vi "Launch Dialog Box.vi"(8 "error in (no error)":errorcluster, 10 "DialogBox":refnum<class "IDialogBox.lvclass">, 11 "IDialogBox in":refnum<class "IDialogBox.lvclass">) -> (0 "error out":errorcluster, 3 "IDialogBox out":refnum<class "IDialogBox.lvclass">)   [LabVIEW 2015, in "IDialogBox.lvlib" / "IDialogBox.lvclass"]
doc: "<License>\nCopyright © 2017 Composed Systems, LLC | All rights reserved\nwww.composed.io\n\nAuthor: Ethan Stern <ethan.stern@composed.io>\n\nThis software is provided \"AS IS\" WITHOUT WARRANTIES, either express or implied, AND IS FOR EDUCATIONAL PURPOSES ONLY.\n</License>"
uses:
  IDialogBox.lvclass
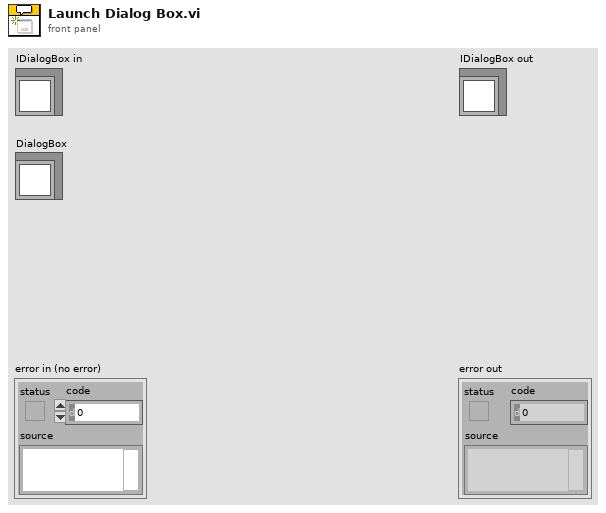
[diagram p1: front panel]
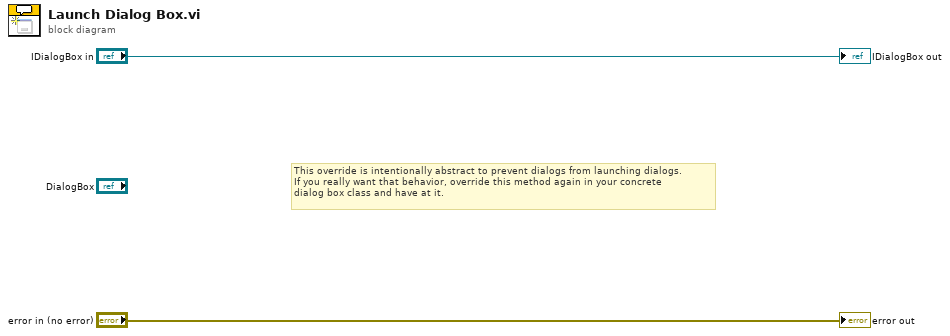
[diagram p0: block diagram]
diagram:
  # "This override is intentionally abstract to prevent dialogs from launching dialogs.\nIf you really want that behavior, override this method again in your concrete\ndialog box class and have at it."
  "error out" <- "error in (no error)"
  "IDialogBox out" <- "IDialogBox in"
